vi "FlatttenMatrix.vi"(1 "Matrix":i32[][](array[numeric])) -> (0 "Array":i32[](array[numeric]))   [LabVIEW 2024]
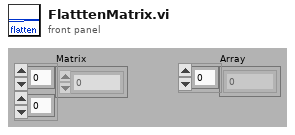
[diagram p1: front panel]
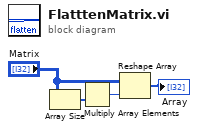
[diagram p0: block diagram]
diagram:
  n1 = Array Size(array="Matrix") -> (size(s)=w2:i32[])
  n2 = Multiply Array Elements(1:w2) -> (0:w1:i32)
  n3 = Reshape Array("Matrix", w1) -> (→"Array":i32[])
